vi "SYST_COMM_GPIB_RDEV_WRIT_ID.vi"(0 "VISA IN":refnum<visa-resource-name>, 1 "Cmd":string, 5 "error in":errorcluster, 7 "ID":i32) -> (14 "VISA Out":refnum<visa-resource-name>, 19 "error out":errorcluster)   [LabVIEW 2018, in "PNA-X.lvlib"]
doc: "SYSTem:COMMunicate:GPIB:RDEVice:WRITe <ID>,<string> \n1872\n\n(Write-only) Sends ASCII string data to the GPIB pass-through device. \nA line feed is NOT appended to the string data. To send a line feed, see the example in \nSYST:COMM:GPIB:RDEV:WBIN. \nParameters \n<ID> Session identification number that was returned with the OPEN? command. \n<string> Commands to be sent to the GPIB pass-through device. \nExamples See an example program \nQuery Syntax Not Applicable \nDefault Not Applicable"
uses:
  PNA-X.lvlib
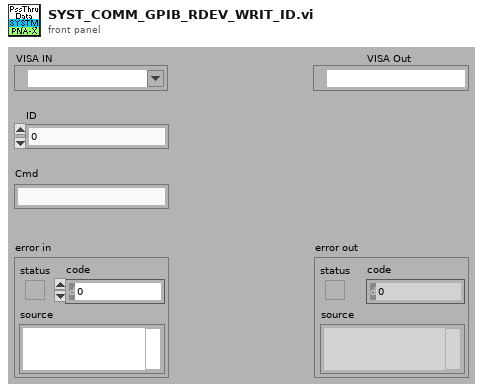
[diagram p1: front panel]
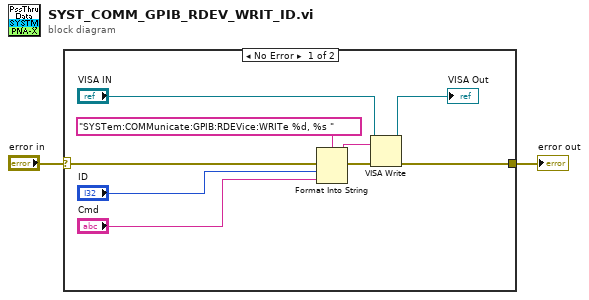
[diagram p0: block diagram]
diagram:
  n1 = case shown="No Error" "error in" {
    selector: "error in" -> [w11 w12]
    tunnel: [w6 w12] -> w1
    frame No Error {
      n2 = Format Into String(format string="SYSTem:COMMunicate:GPIB:RDEVice:WRITe %d, %s " ("Cmdline"), error in=w11, "ID", "Cmd") -> (resulting string=w9:string, error out=w10:errorcluster)  [unwired: 1 in]
      n3 = VISA Write(VISA resource name="VISA IN", write buffer=w9, error in (no error)=w10) -> (VISA resource name out=→"VISA Out":refnum<visa-resource-name>, error out=w6:errorcluster)  [unwired: 1 out]
    }
    frame Error {
    }
  }
  "error out" <- w1
